vi "Page_Source_Configure_TopVI.vi"(8 "error in (no error)":errorcluster, 11 "AB_Source_ExportedVI in":refnum<class "AB_Source_ExportedVI.lvclass">) -> (0 "error out":errorcluster, 2 "cancelled":bool, 3 "AB_Source_ExportedVI out":refnum<class "AB_Source_ExportedVI.lvclass">)   [LabVIEW 2020, in "AB_Source_ExportedVI.lvclass"]
uses:
  <vilib>/AppBuilder/AB_Classes/Source/ExportedVI/AB_Source_ExportedVI.lvclass
  e:/builds/penguin/labview/branches/2020/dev/dist/vi.lib/AppBuilder/AB_Classes/Source/AB_Source.lvclass
  <vilib>/AppBuilder/AB_Classes/Source/ExportedVI/AB_Source_ExportedVI.lvclass/AB_Source_ExportedVI.ctl
  <vilib>/AppBuilder/ABAPI Dist VI Proto Info New.ctl
  <resource>/Framework/Providers/Common/provcom_StringGlobals.vi
  <vilib>/AppBuilder/AB_Classes/Build/AB_Build.lvclass
  <vilib>/AppBuilder/AB_Classes/Source/AB_Source.lvclass
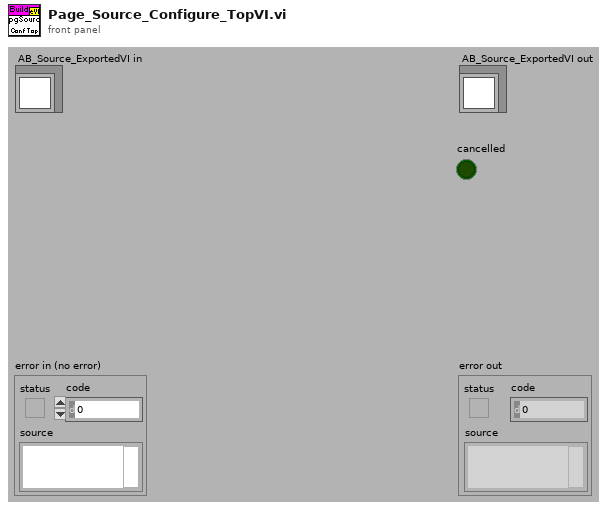
[diagram p1: front panel]
types:
  T1 = typedef "AB_Source.ctl" = cluster{"path":path, "itemID":string, "parentIndex":i32, "sourceInclusion":T2, "destinationIndex":i32, "properties":T3[], "newName":string, "lvfile":bool, "valid":bool, "eng_inBuild":bool, "eng_isNonVILink":bool, "Amalgamation":bool, "Amalgamation Piece":bool, "eng_delimitedName":string, "preventRename":bool}
  T2 = typedef "AB_Source_Inclusion.ctl" = enum16{"IncludeIfReferenced", "Include", "Exclude", "TopLevel"}
  T3 = typedef "AB_Source_Properties.ctl" = cluster{"sourcePropertyType":T4, "value":variant}
  T4 = typedef "AB_Source_Property_Type.ctl" = enum16{"Remove block diagram", "Remove front panel", "Password", "Window has title bar", "Show menu bar", "Show vertical scroll bar", "Show horizontal scroll bar", "Show toolbar", "Show Abort button", "Show fp when called", "Window behavior", "Allow user to close window", "Window run-time position", "Run when opened", "Allow debugging", "Auto error handling", "Generate guard code", "Use stack variables", "Expression folding", "Integer only", "Inline subVI"}
  T5 = typedef "ABAPI Dist VI Proto Info New.ctl" = cluster{"cptm":string, "params":cluster{"name":string, "dir":enum32{"in", "out", "in/out", "length", "error-out"}, "inputIdx":i32, "outputIdx":i32, "passBy":i32, "lenInput":i32, "lenOutput":i32}[], "callingConv":i32, "name":string, "Description":string, "isCustomDesc":i32}
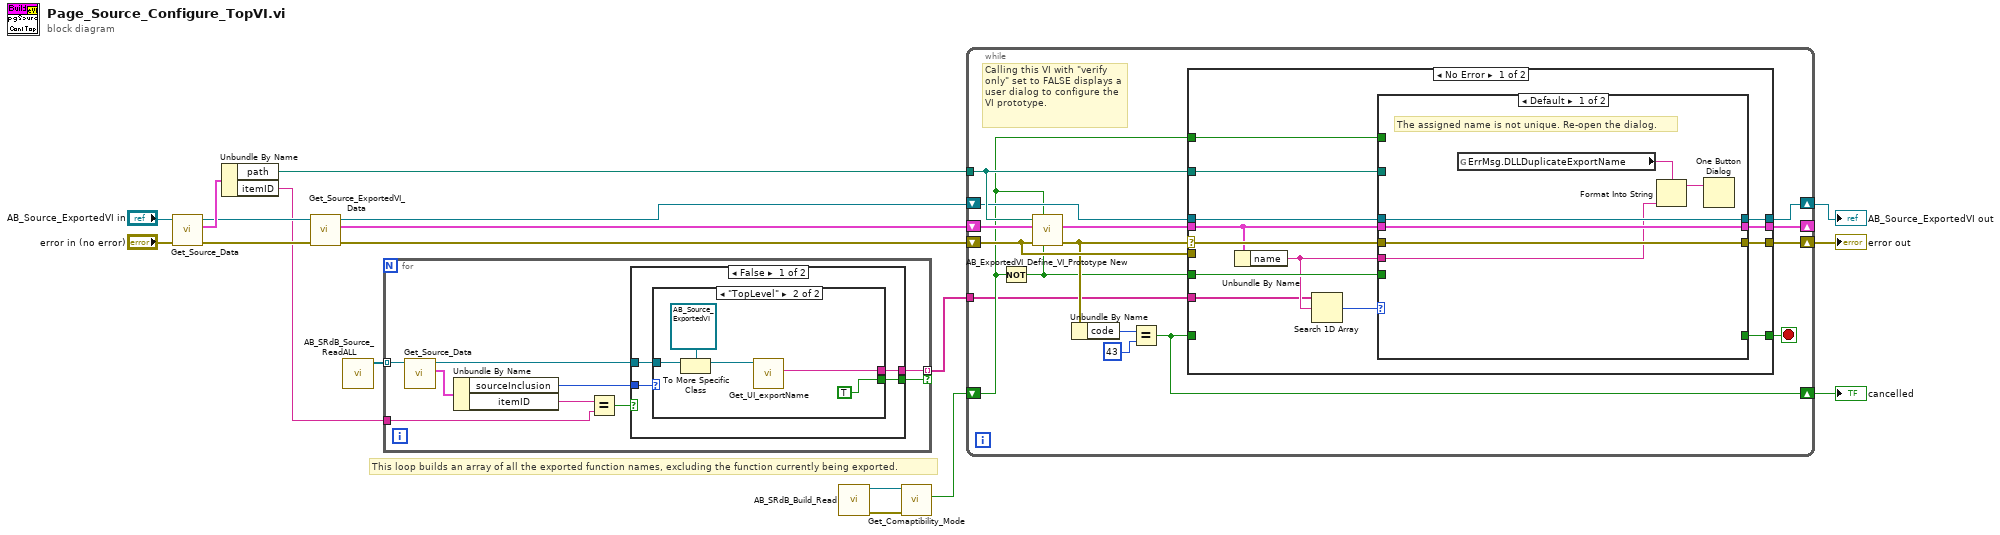
[diagram p0: block diagram]
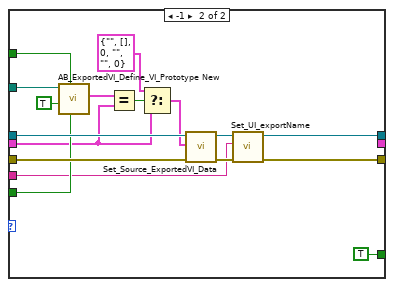
[diagram p2: hidden frame]
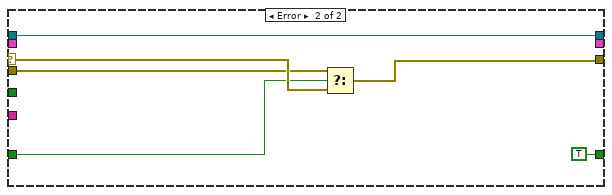
[diagram p3: hidden frame]
diagram:
  # "This loop builds an array of all the exported function names, excluding the function currently being exported."
  n1 = call <vilib>:"Get_Source_Data.vi"("error in (no error)"="error in (no error)", "Class in"="AB_Source_ExportedVI in") -> ("error out"=w13:errorcluster, "data"=w17:T1, "Class out"=w12:refnum<class "AB_Source_ExportedVI.lvclass">)  [unwired: 7 in]
  n2 = Unbundle By Name(w17) -> ("path"=w18:path, "itemID"=w2:string)
  n3 = call <vilib>:"Get_Source_ExportedVI_Data.vi"("error in (no error)"=w13, "Class in"=w12) -> ("error out"=w14:errorcluster, "data"=w15:T5, "Class out"=w16:refnum<class "AB_Source_ExportedVI.lvclass">)  [unwired: 7 in]
  n4 = call <resource>:"AB_SRdB_Source_ReadALL.vi"() -> ("ALL data"=w3:refnum<class "AB_Source.lvclass">[])  [unwired: 10 in, 1 out]
  n5 = for {
    tunnel: w3 -> [w27] mode=indexing
    tunnel: [w23] -> w1 mode=indexing if=w22
    tunnel: w2 -> [w21]
    n6 = call <vilib>:"Get_Source_Data.vi"("Class in"=w27) -> ("data"=w26:T1, "Class out"=w25:refnum<class "AB_Source.lvclass">)  [unwired: 8 in, 1 out]
    n7 = Unbundle By Name(w26) -> ("sourceInclusion"=w24:T2, "itemID"=w20:string)
    n8 = Equal?(x=w20, y=w21) -> (x = y?=w19:bool)
    n9 = case shown="False" w19 {
      tunnel: w25 -> [w31 _]
      tunnel: w24 -> [w30 _]
      tunnel: [w29 _] -> w23
      tunnel: [w28 _] -> w22
      frame False {
        n10 = case shown="\"TopLevel\"" w30 {
          tunnel: w31 -> [_ w35]
          tunnel: [_ w32] -> w29
          tunnel: [_ TRUE] -> w28
          frame Default {
          }
          frame "TopLevel" {
            n11 = To More Specific Class(target class=refnum<class "AB_Source_ExportedVI.lvclass"> refnum ("Class out"), reference=w35) -> (specific class reference=w33:refnum<class "AB_Source_ExportedVI.lvclass">)  [unwired: 1 in, 1 out]
            n12 = call <vilib>:"Get_UI_exportName.vi"("AB_Source_ExportedVI in"=w33) -> ("UI_exportName"=w32:string)  [unwired: 8 in, 2 out]
          }
        }
      }
      frame True {
        # "do not add the file we're checking to the list"
      }
    }
  }
  n13 = call <resource>:"AB_SRdB_Build_Read.vi"() -> ("error out"=w5:errorcluster, "build out"=w6:refnum<class "AB_Build.lvclass">)  [unwired: 10 in]
  n14 = call-dynamic "Get_Comaptibility_Mode.vi"("error in (no error)"=w5, "AB_Build in"=w6) -> ("CompatibilityWith2011"=w4:bool)  [unwired: 7 in, 2 out]
  n15 = while {
    tunnel: w18 -> [w52]
    tunnel: w1 -> [w40]
    shift-right: [w46] -> w7
    shift-left: w16 -> [w51]
    shift-right: [w47] -> w9
    shift-left: w14 -> [w49]
    shift-right: [w37] -> w11
    shift-left: w4 -> [w45]
    shift-right: [w38] -> _
    shift-left: w15 -> [w50]
    stop <- w39 stop-if-true
    # "Calling this VI with \"verify only\" set to FALSE displays a user dialog to configure the VI prototype."
    n16 = Not(x=w45) -> (.not. x?=w44:bool)
    n17 = call <vilib>:"AB_ExportedVI_Define_VI_Prototype New.vi"("generateNamespace"=w44, "compatibilityMode"=w45, "error in (no error)"=w49, "vipInfo in"=w50, "path"=w52) -> ("error out"=w48:errorcluster, "vipInfo out"=w43:T5)  [unwired: 4 in, 1 out]
    n18 = Unbundle By Name(w48) -> ("code"=w42:i32)
    n19 = Equal?(x=w42, y=43) -> (x = y?=w37:bool)
    n20 = case shown="No Error" w48 {
      selector: w48 -> [w64 w93]
      tunnel: w43 -> [w58 _]
      tunnel: w51 -> [w65 w91]
      tunnel: [w59 w94] -> w47
      tunnel: w49 -> [_ w92]
      tunnel: w37 -> [_ w90]
      tunnel: w52 -> [w63 _]
      tunnel: [w60 w91] -> w46
      tunnel: w45 -> [w62 _]
      tunnel: w44 -> [w61 _]
      tunnel: w40 -> [w56 _]
      tunnel: [w54 TRUE] -> w39
      tunnel: [w53 _] -> w38
      frame No Error {
        n21 = Unbundle By Name(w58) -> ("name"=w57:string)
        n22 = Search 1D Array(1D array=w56, element=w57) -> (index of element=w55:i32)  [unwired: 1 in]
        n23 = case shown="Default" w55 {
          tunnel: w65 -> [w71 w88]
          tunnel: w64 -> [w70 w87]
          tunnel: w63 -> [_ w84]
          tunnel: w62 -> [_ w80]
          tunnel: w61 -> [_ w79]
          tunnel: [w71 w77] -> w60
          tunnel: [w70 w75] -> w59
          tunnel: w58 -> [w69 w74]
          tunnel: w57 -> [w66 w73]
          tunnel: [_ TRUE] -> w54
          tunnel: [w69 _] -> w53
          frame Default {
            # "The assigned name is not unique. Re-open the dialog."
            n24 = global read "provcom_StringGlobals.vi" "ErrMsg.DLLDuplicateExportName"() -> (w68:string)
            n25 = Format Into String(format string=w68, w66) -> (resulting string=w67:string)  [unwired: 2 in, 1 out]
            n26 = One Button Dialog(message=w67) -> ()  [unwired: 1 in, 1 out]
          }
          frame -1 {
            n27 = call <vilib>:"AB_ExportedVI_Define_VI_Prototype New.vi"("generateNamespace"=w79, "compatibilityMode"=w80, "verify only"=TRUE, "path"=w84) -> ("vipInfo out"=w86:T5)  [unwired: 5 in, 2 out]
            n28 = Equal?(x=w86, y=w74) -> (x = y?=w83:bool)
            n29 = Select(t=T5 {"cptm"="", "params"=[], "callingConv"=0, "name"="", "Description"="", "isCustomDesc"=0} ("vipInfo in"), s=w83, f=w74) -> (s? t:f=w82:T5)
            n30 = call <vilib>:"Set_Source_ExportedVI_Data.vi"("error in (no error)"=w87, "data"=w82, "Class in"=w88) -> ("error out"=w76:errorcluster, "Class out"=w78:refnum<class "AB_Source_ExportedVI.lvclass">)  [unwired: 7 in]
            n31 = call <vilib>:"Set_UI_exportName.vi"("error in (no error)"=w76, "UI_exportName"=w73, "AB_Source_ExportedVI in"=w78) -> ("error out"=w75:errorcluster, "AB_Source_ExportedVI out"=w77:refnum<class "AB_Source_ExportedVI.lvclass">)  [unwired: 7 in]
          }
        }
      }
      frame Error {
        n32 = Select(t=w92, s=w90, f=w93) -> (s? t:f=w94:errorcluster)
      }
    }
  }
  "error out" <- w9
  "AB_Source_ExportedVI out" <- w7
  "cancelled" <- w11
